vi "UpdateLibApperance.vi"(0 "LibRefIn":refnum<vi>, 2 "MessageClass(False)":bool, 5 "error in (no error)":errorcluster) -> (14 "LibRefOut":refnum<vi>, 19 "error out":errorcluster)   [LabVIEW 2014, in "LibWriter.lvclass"]
uses:
  <resource>/Framework/Providers/Open_GDS/ClassProviders/LibProvider_BaseClassInterface/LibWriter_class/ClassWriter_class/LibWriter.lvclass
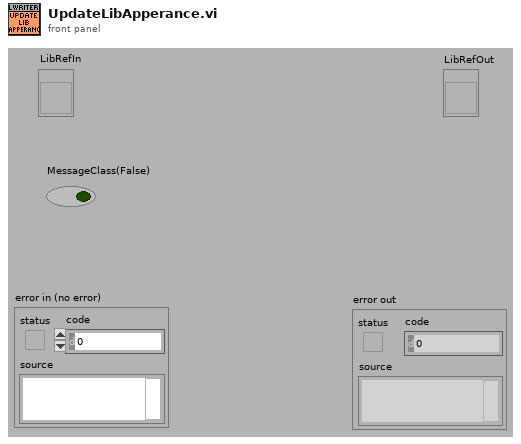
[diagram p1: front panel]
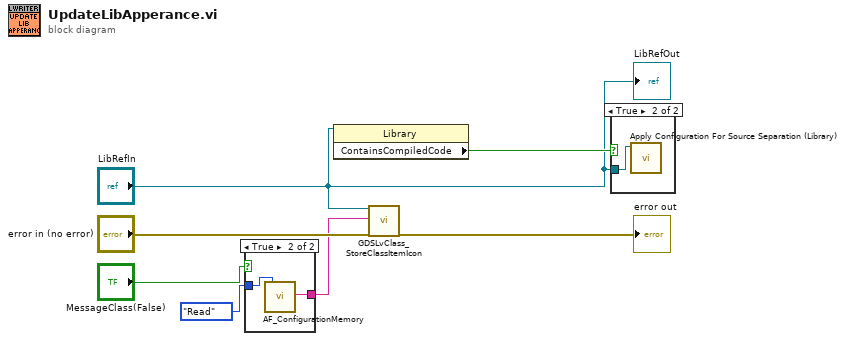
[diagram p0: block diagram]
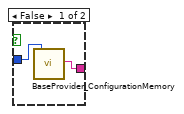
[diagram p3: hidden frame]
diagram:
  n1 = case shown="True" "MessageClass(False)" {
    tunnel: [w9 w10] -> w5
    tunnel: enum16{"Read", "Load", "Save", "Set"}."Read" ("Action") -> [w8 w11]
    frame False {
      n2 = call <resource>:"BaseProvider_ConfigurationMemory.vi"("Action"=w8) -> ("IconOut"=w9:string)  [unwired: 12 in, 6 out]
    }
    frame True {
      n3 = call <resource>:"AF_ConfigurationMemory.vi"("Action"=w11) -> ("IconOut"=w10:string)  [unwired: 15 in, 3 out]
    }
  }
  n4 = property class="Library"(reference="LibRefIn") -> ("ContainsCompiledCode"=w2:bool)  [unwired: 1 in, 2 out]
  n5 = call <resource>:"GDSLvClass_StoreClassItemIcon.vi"("Library Refnum"="LibRefIn", "ClassItemIconName"=w5, "error in (no error)"="error in (no error)") -> ("error out"=→"error out":errorcluster)  [unwired: 15 in, 1 out]
  n6 = case shown="True" w2 {
    tunnel: "LibRefIn" -> [_ w12]
    frame False {
    }
    frame True {
      n7 = call <vilib>:"Apply Configuration For Source Separation (Library).vi"("Library in"=w12) -> ()  [unwired: 9 in, 2 out]
    }
  }
  "LibRefOut" <- "LibRefIn"
